vi "MaquinaDeEstados.vi"() -> ()   [LabVIEW 2025]
panel:
  out "Se;ñal timer activa":bool
  out "Se;ñal timer":bool
  out "V3":bool
  out "V2":bool
  out "V1":bool
  out "VB":bool
  out "VA":bool
  out "Estado":u32
  out "Motor activo":bool
  in  "stop":bool
  in  "DU":bool
  in  "DL":bool
  in  "SP2":bool
  in  "SP1":bool
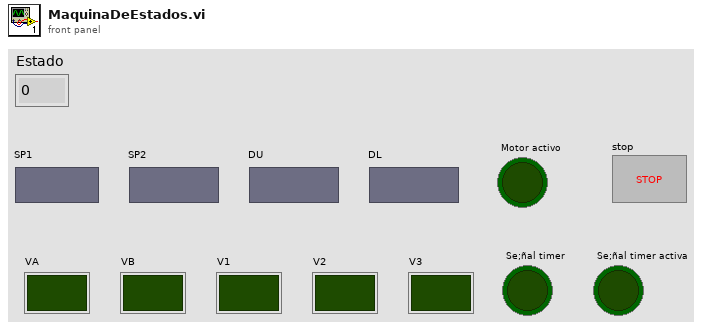
[diagram p1: front panel]
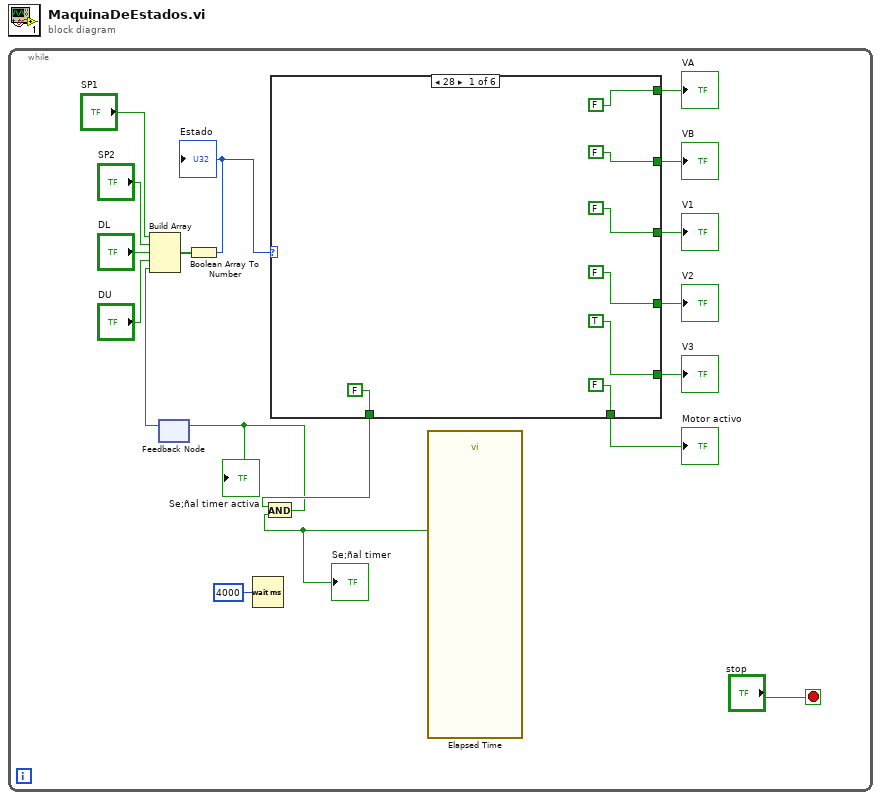
[diagram p0: block diagram]
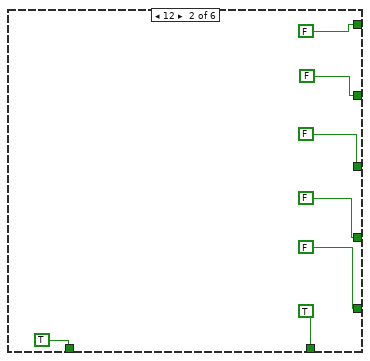
[diagram p2: hidden frame]
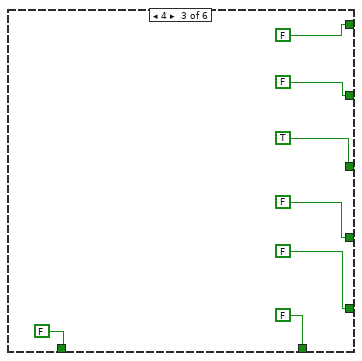
[diagram p3: hidden frame]
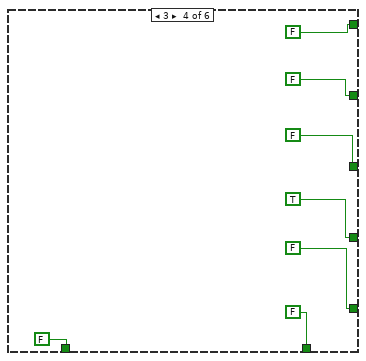
[diagram p4: hidden frame]
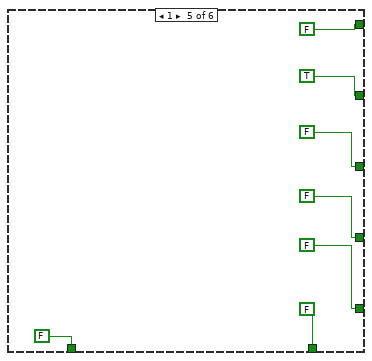
[diagram p5: hidden frame]
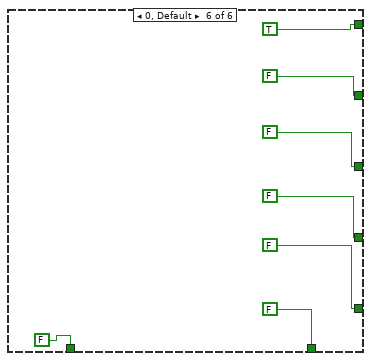
[diagram p6: hidden frame]
diagram:
  n1 = while {
    stop <- "stop" stop-if-true
    n2 = feedback #1() -> (w3:bool)  [unwired: 1 in]
    n3 = Build Array("SP1", "SP2", "DL", "DU", w3) -> (w13:bool[])
    n4 = Boolean Array To Number(Boolean array=w13) -> (number=w12:u32)
    "Estado" <- w12
    n5 = Wait (ms)(milliseconds to wait=u32 4000) -> ()  [unwired: 1 out]
    n6 = case shown="28" w12 {
      tunnel: [FALSE ("Auto Reset") FALSE ("Auto Reset") FALSE ("Auto Reset") FALSE ("Auto Reset") FALSE ("Auto Reset") TRUE ("Auto Reset")] -> w11
      tunnel: [FALSE ("Auto Reset") FALSE ("Auto Reset") FALSE ("Auto Reset") FALSE ("Auto Reset") TRUE ("Auto Reset") FALSE ("Auto Reset")] -> w10
      tunnel: [FALSE ("Auto Reset") FALSE ("Auto Reset") TRUE ("Auto Reset") FALSE ("Auto Reset") FALSE ("Auto Reset") FALSE ("Auto Reset")] -> w9
      tunnel: [FALSE ("Auto Reset") FALSE ("Auto Reset") FALSE ("Auto Reset") TRUE ("Auto Reset") FALSE ("Auto Reset") FALSE ("Auto Reset")] -> w8
      tunnel: [TRUE ("Auto Reset") FALSE ("Auto Reset") FALSE ("Auto Reset") FALSE ("Auto Reset") FALSE ("Auto Reset") FALSE ("Auto Reset")] -> w7
      tunnel: [FALSE ("Auto Reset") TRUE ("Auto Reset") FALSE ("Auto Reset") FALSE ("Auto Reset") FALSE ("Auto Reset") FALSE ("Auto Reset")] -> w6
      tunnel: [FALSE ("Auto Reset") TRUE ("Auto Reset") FALSE ("Auto Reset") FALSE ("Auto Reset") FALSE ("Auto Reset") FALSE ("Auto Reset")] -> w4
      frame 28 {
      }
      frame 12 {
      }
      frame 4 {
      }
      frame 3 {
      }
      frame 1 {
      }
      frame 0, Default {
      }
    }
    "Motor activo" <- w6
    "VA" <- w11
    "V1" <- w9
    "V2" <- w8
    "V3" <- w7
    "VB" <- w10
    n7 = call "Elapsed Time"() -> ("Time has Elapsed"=w5:bool)  [unwired: 12 in, 7 out]
    "Se;ñal timer" <- w5
    n8 = And(x=w4, y=w5) -> (x .and. y?=w1:bool)
    "Se;ñal timer activa" <- w1
    n9 = feedback-in #1(w1) -> ()
  }
